vi "yaqd_status.vi"(10 "Python path":path=path "C:/ProgramData/Anaconda3/envs/lv4/pythonw.exe") -> (0 "error out":errorcluster, 4 "yaqd status cluster":T1)   [LabVIEW 2022 SP3]
doc: "Returns the statuses of daemons available, as host, port, kind, name, status, and busy. These arrays can then be searched using array VIs."
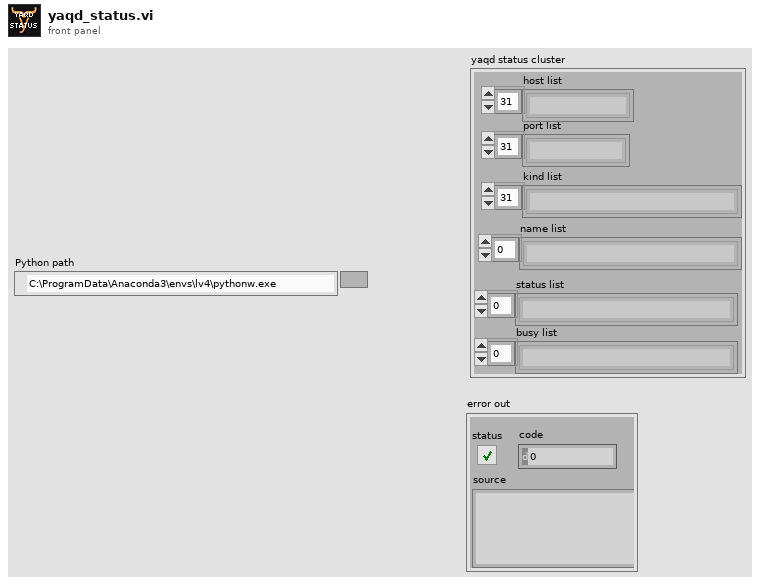
[diagram p1: front panel]
types:
  T1 = cluster{"host list":string[], "port list":string[], "kind list":string[], "name list":string[], "status list":string[], "busy list":string[]}
  T2 = cluster{string[], string[], string[], string[], string[], string[]}
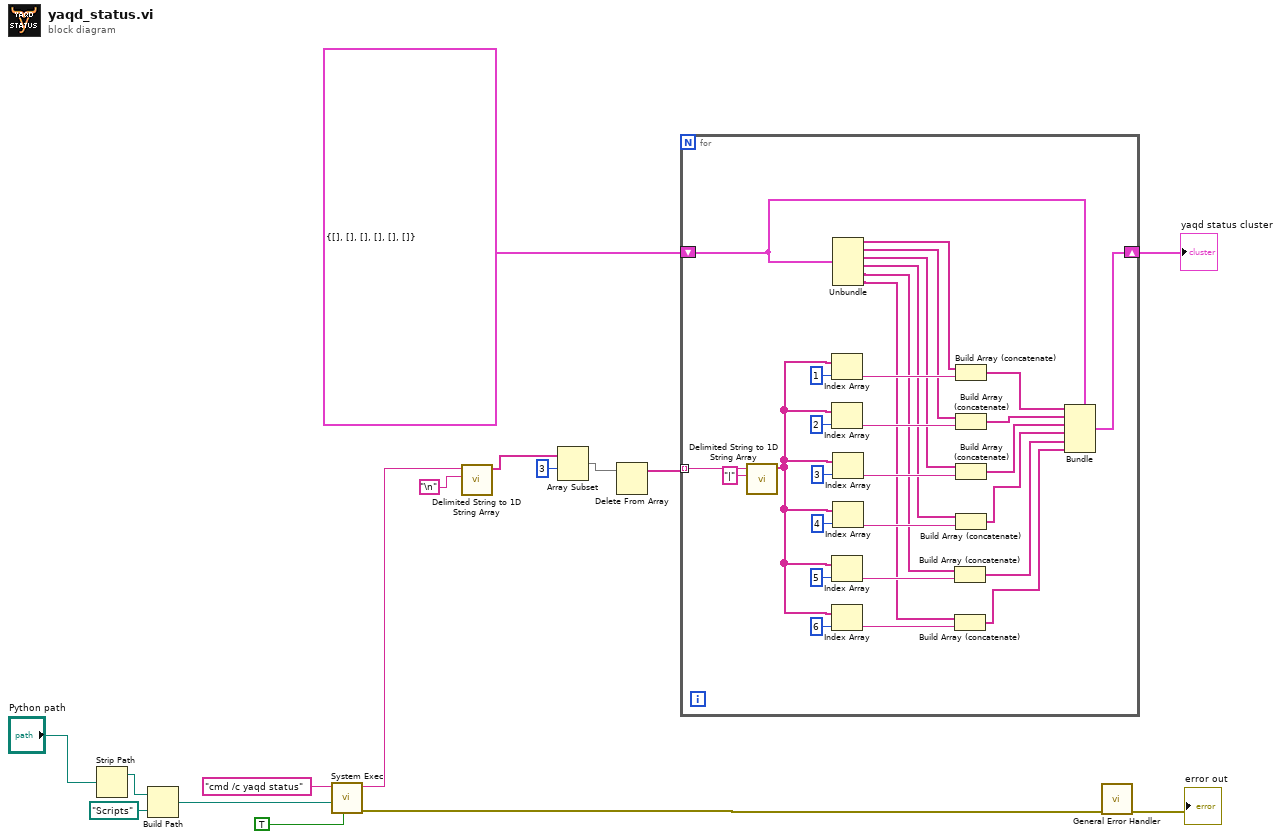
[diagram p0: block diagram]
diagram:
  n1 = Strip Path(path="Python path") -> (stripped path=w13:path)  [unwired: 1 out]
  n2 = Build Path(base path=w13, name or relative path=path "Scripts") -> (appended path=w10:path)
  n3 = call <vilib>:"System Exec.vi"("run minimized? (F)"=TRUE, "working directory"=w10, "command line"="cmd /c yaqd status") -> ("error out"=w15:errorcluster, "standard output"=w8:string)  [unwired: 5 in, 2 out]
  n4 = call <vilib>:"Delimited String to 1D String Array.vi"("delimiter"="\n", "delimited string"=w8) -> ("string array"=w4:string[])  [unwired: 9 in]
  n5 = Array Subset(array=w4, index=3) -> (w2:string[])  [unwired: 1 in]
  n6 = Delete From Array(array=w2) -> (array with subset deleted=w1:string[])  [unwired: 2 in, 1 out]
  n7 = for {
    tunnel: w1 -> [w45] mode=indexing
    shift-right: [w26] -> w5
    shift-left: T2 {[], [], [], [], [], []} -> [w27]
    n8 = call <vilib>:"Delimited String to 1D String Array.vi"("delimiter"="|", "delimited string"=w45) -> ("string array"=w19:string[])  [unwired: 9 in]
    n9 = Index Array(array=w19, index=1) -> (element=w39:string)
    n10 = Index Array(array=w19, index=2) -> (element=w38:string)
    n11 = Index Array(array=w19, index=5) -> (element=w24:string)
    n12 = Index Array(array=w19, index=6) -> (element=w25:string)
    n13 = Unbundle(w27) -> (w35:string[], w34:string[], w33:string[], w32:string[], w18:string[], w17:string[])
    n14 = Index Array(array=w19, index=3) -> (element=w37:string)
    n15 = Index Array(array=w19, index=4) -> (element=w36:string)
    n16 = Build Array (concatenate)(w18, w24) -> (w21:string[])
    n17 = Build Array (concatenate)(w17, w25) -> (w20:string[])
    n18 = Build Array (concatenate)(w35, w39) -> (w31:string[])
    n19 = Build Array (concatenate)(w34, w38) -> (w30:string[])
    n20 = Build Array (concatenate)(w33, w37) -> (w29:string[])
    n21 = Build Array (concatenate)(w32, w36) -> (w28:string[])
    n22 = Bundle(cluster=w27, w31, w30, w29, w28, w21, w20) -> (w26:T2)
  }
  "yaqd status cluster" <- w5
  n23 = call <vilib>:"General Error Handler.vi"("error in (no error)"=w15) -> ("error out"=→"error out":errorcluster)  [unwired: 10 in, 4 out]
